vi "Get Message Type.vi"(8 "error in":errorcluster, 11 "message in":T2 format="%.0x") -> (0 "error out":errorcluster, 2 "message type":T1, 3 "message out":T2 format="%.0x", 4 "found?":bool)   [LabVIEW 2020, in "Ballard MIL-STD-1553 Scripting.lvlib"]
doc: "Reads the <b>description</b> field of the input <b>Ballard MIL-STD 1553 custom device</b>."
uses:
  <vilib>/NI VeriStand/Custom Device API/Custom Device Item Ref.ctl
  Constants.vi
  <vilib>/NI VeriStand/Custom Device API/Get Item Property (String).vi
  Ballard MIL-STD-1553 Scripting.lvlib
  <vilib>/NI VeriStand/Custom Device API/Custom Device API.lvlib
  Shared/Message Type.ctl
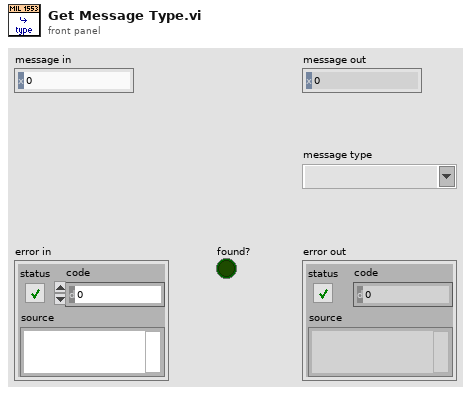
[diagram p1: front panel]
types:
  T1 = typedef "Message Type.ctl" = string
  T2 = typedef "Custom Device API.lvlib/Custom Device Item Ref.ctl" = u64
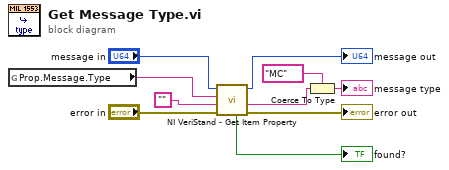
[diagram p0: block diagram]
diagram:
  n1 = global read "Constants.vi" "Prop.Message.Type"() -> (w5:string)
  n2 = call-poly <vilib>:"NI VeriStand - Get Item Property.vi"("error in (no error)"="error in", "Default Value"="", "Property Name"=w5, "Item Ref in"="message in") -> ("error out"=→"error out":errorcluster, "Value"=w2:string, "Item Ref out"=→"message out":T2, "Found?"=→"found?":bool)  [unwired: 4 in]
  n3 = Coerce To Type(0:w2, 1:T1 "MC" ("message type")) -> (2:→"message type":T1)
